vi "Mouse click event.vi"() -> ()   [LabVIEW 2018]
panel:
  out "No of times clicked":dbl(slide) scale=0.0..10.0
  in  "Click":bool
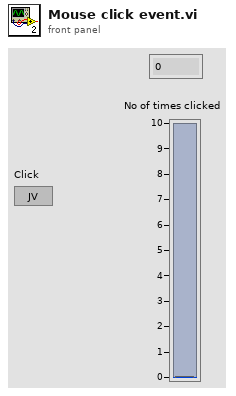
[diagram p1: front panel]
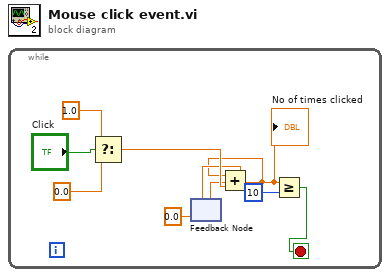
[diagram p0: block diagram]
diagram:
  n1 = while {
    stop <- w9 stop-if-true
    n2 = Select(t=1.0, s="Click", f=0.0) -> (s? t:f=w4:dbl)
    n3 = feedback #1(0.0) -> (w1:dbl)
    "No of times clicked" <- w1
    n4 = Add(x=w1, y=w4) -> (x+y=w3:dbl)
    n5 = feedback-in #1(w3) -> ()
    n6 = Greater Or Equal?(x=w1, y=10) -> (x >= y?=w9:bool)
  }
